vi "init.vi"(8 "error in (no error)":errorcluster, 11 "Application in":refnum<class "Application.lvclass">) -> (0 "error out":errorcluster, 3 "Application out":refnum<class "Application.lvclass">)   [LabVIEW 2013, in "Application.lvlib" / "Application.lvclass"]
uses:
  <userlib>/Common/Component/Application/Application/Application.lvclass
  <userlib>/Common/Component/Application/Configuration/Application.ctl
  <userlib>/Common/Component/Application/Application/Application.lvclass/Application.ctl
  <userlib>/Common/Component/Application/Application.lvlib
  LSST_TS/SystemSW/M2AADT/ConfigurationThisComponent/ConfigurationThisComponent.lvclass
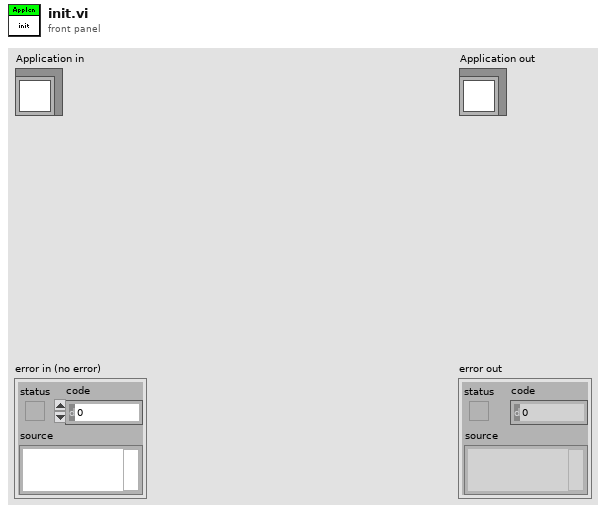
[diagram p1: front panel]
types:
  T1 = typedef "Application.lvlib/Application.ctl" = cluster{"Loop Period (ms)":u16}
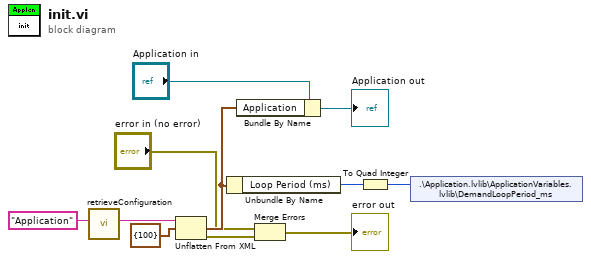
[diagram p0: block diagram]
diagram:
  n1 = call "retrieveConfiguration.vi"("configName"="Application") -> ("xmlConfig"=w1:string)  [unwired: 8 in, 2 out]
  n2 = Unflatten From XML(xml string=w1, type=T1 {"Loop Period (ms)"=100} ("Application Timing")) -> (value=w4:T1, error out=w10:errorcluster)  [unwired: 1 in]
  n3 = Unbundle By Name(w4) -> ("Loop Period (ms)"=w6:u16)
  n4 = Bundle By Name(cluster="Application in", "Application"=w4) -> (→"Application out":refnum<class "Application.lvclass">)
  n5 = Merge Errors("error in (no error)", w10) -> (→"error out":errorcluster)
  n6 = To Quad Integer(1:w6) -> (0:w5:i64)
  n7 = shared-variable ".\\Application.lvlib\\ApplicationVariables.lvlib\\DemandLoopPeriod_ms"(w5) -> ()  [unwired: 1 in, 1 out]
